vi "Read Currency.vi"() -> (0 "error out":errorcluster, 3 "Array":cluster{"Denomination":string, "Value":dbl}[](array[cluster]))   [LabVIEW 2020, in "Config File Management.lvlib"]
doc: "Reads the infromation in the config file and returns an array of clusters with the information for every coin."
uses:
  Config File Management.lvlib
  <vilib>/Utility/config.llb/Read Key (String).vi
  <vilib>/Utility/config.llb/Read Key (Double).vi
  <vilib>/Utility/config.llb/NI_LVConfig.lvlib
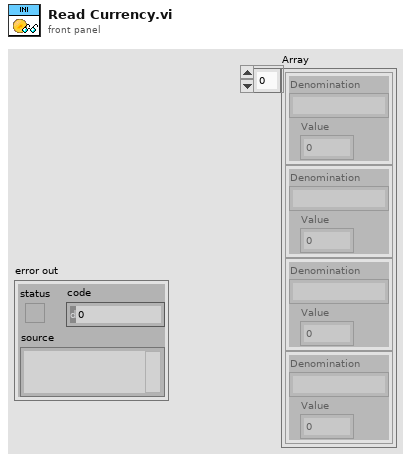
[diagram p1: front panel]
types:
  T1 = typedef "NI_LVConfig.lvlib/Config Data RefNum.ctl" = refnum<k1>
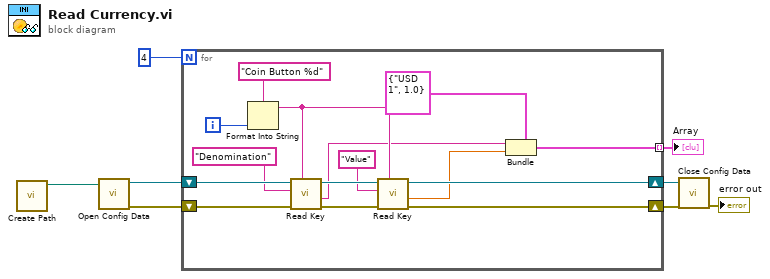
[diagram p0: block diagram]
diagram:
  n1 = call "Create Path.vi"() -> ("Config File path"=w4:path)  [unwired: 11 in]
  n2 = call <vilib>:"Open Config Data.vi"("configuration file path"=w4) -> ("error out"=w8:errorcluster, "refnum"=w7:T1)  [unwired: 8 in, 1 out]
  n3 = for {
    N: 4 -> [_]
    shift-right: [w20] -> w5
    shift-left: w8 -> [w23]
    shift-right: [w17] -> w6
    shift-left: w7 -> [w22]
    tunnel: [w12] -> w1 mode=indexing
    i -> [w9]
    n4 = Format Into String(format string="Coin Button %d", w9) -> (resulting string=w16:string)  [unwired: 2 in, 1 out]
    n5 = call-poly <vilib>:"Read Key.vi"("section"=w16, "error in (no error)"=w23, "key"="Denomination", "refnum"=w22) -> ("error out"=w19:errorcluster, "value"=w11:string, "refnum out"=w18:T1)  [unwired: 4 in, 1 out]
    n6 = call-poly <vilib>:"Read Key.vi"("section"=w16, "error in (no error)"=w19, "key"="Value", "refnum"=w18) -> ("error out"=w20:errorcluster, "value"=w10:dbl, "refnum out"=w17:T1)  [unwired: 4 in, 1 out]
    n7 = Bundle(cluster=cluster{"Denomination":string, "Value":dbl} {"Denomination"="USD 1", "Value"=1.0} ("Coin"), "Denomination"=w11, "Value"=w10) -> (w12:cluster{"Denomination":string, "Value":dbl})
  }
  "Array" <- w1
  n8 = call <vilib>:"Close Config Data.vi"("error in (no error)"=w5, "refnum"=w6) -> ("error out"=→"error out":errorcluster)  [unwired: 8 in, 1 out]
